vi "svfa_Check for FRF Mode Change (Dual).vi"(4 "measurement":T1(ring), 6 "FRF mode":enum16{"H1", "H2", "H3"}(ring), 7 "restart":bool, 8 "error in (no error)":errorcluster) -> (0 "error out":errorcluster, 1 "parameter has changed":bool)   [LabVIEW 2017]
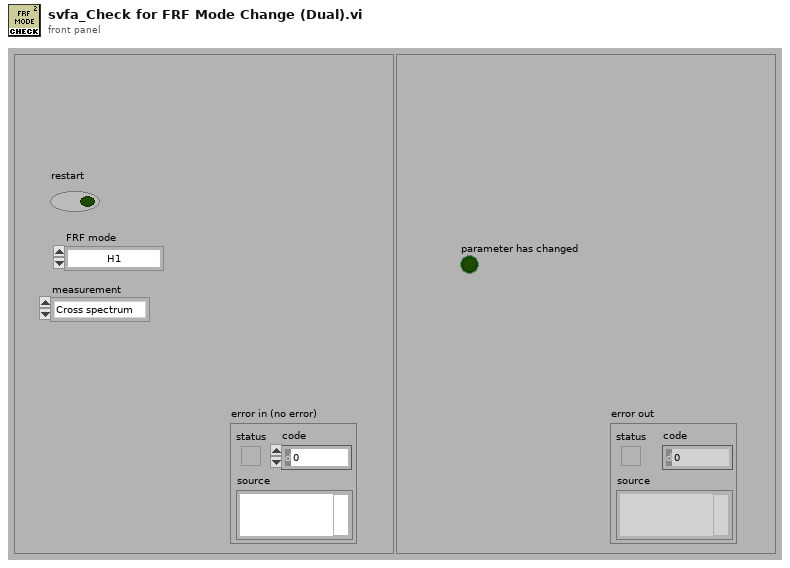
[diagram p1: front panel]
types:
  T1 = enum16{"Cross spectrum", "Frequency response", "Coherent output power"}
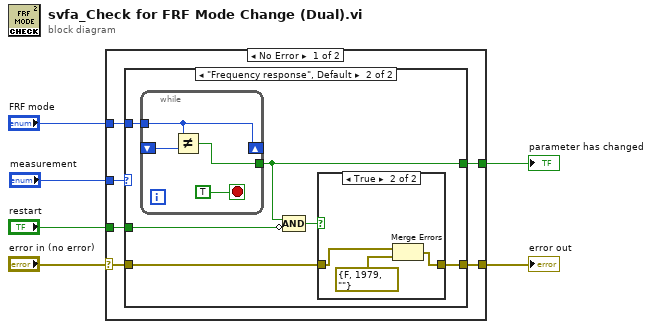
[diagram p0: block diagram]
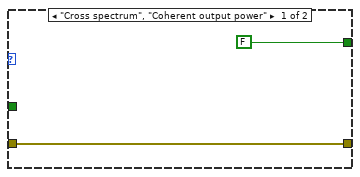
[diagram p2: hidden frame]
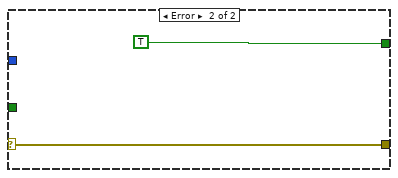
[diagram p4: hidden frame]
diagram:
  n1 = case shown="No Error" "error in (no error)" {
    selector: "error in (no error)" -> [w9 w30]
    tunnel: [w12 TRUE] -> w6
    tunnel: "FRF mode" -> [w11 _]
    tunnel: [w8 w30] -> w3
    tunnel: "measurement" -> [w10 _]
    tunnel: "restart" -> [w7 _]
    frame No Error {
      n2 = case shown="\"Frequency response\", Default" w10 {
        tunnel: [FALSE w15] -> w12
        tunnel: w11 -> [_ w20]
        tunnel: w9 -> [w13 w19]
        tunnel: [w13 w18] -> w8
        tunnel: w7 -> [_ w17]
        frame "Cross spectrum", "Coherent output power" {
        }
        frame "Frequency response", Default {
          n3 = while {
            tunnel: [w21] -> w15
            tunnel: w20 -> [w22]
            shift-left: _ -> [w23]
            shift-right: [w22] -> _
            stop <- TRUE stop-if-true
            n4 = Not Equal?(x=w22, y=w23) -> (x != y?=w21:bool)
          }
          n5 = Compound Arithmetic op=AND(w15, invert w17) -> (w16:bool)
          n6 = case shown="True" w16 {
            tunnel: w19 -> [w25 w28]
            tunnel: [w25 w26] -> w18
            frame False {
            }
            frame True {
              n7 = Merge Errors(w28, errorcluster {"status"=FALSE, "code"=1979, "source"=""} ("error IO")) -> (w26:errorcluster)
            }
          }
        }
      }
    }
    frame Error {
    }
  }
  "error out" <- w3
  "parameter has changed" <- w6
